vi "Parse Frequencies.vi"(0 "Frequencies in":string[](array[string]), 11 "error in (no error)":errorcluster) -> (4 "Frequencies out":dbl[](array[numeric]), 15 "error out":errorcluster)   [LabVIEW 2023, in "RFCalAndFixtureCharact.Common.lvlib"]
uses:
  RFCalAndFixtureCharact.Common.lvlib
  <vilib>/regexp/Match Regular Expression.xnode
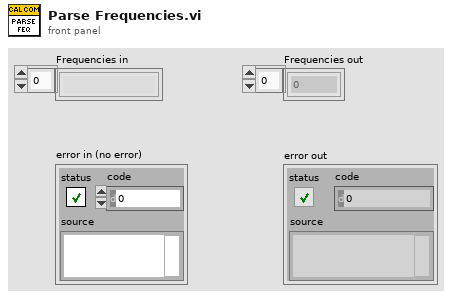
[diagram p1: front panel]
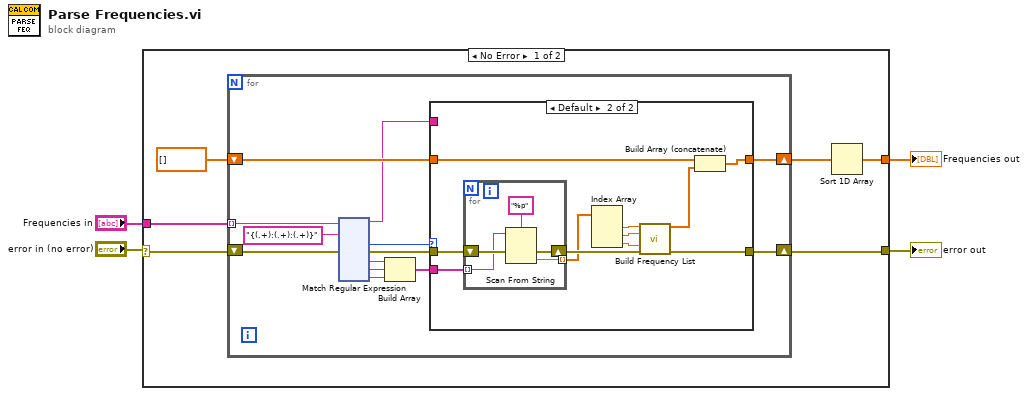
[diagram p0: block diagram]
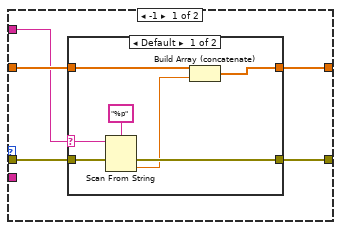
[diagram p2: hidden frame]
diagram:
  n1 = case shown="No Error" "error in (no error)" {
    selector: "error in (no error)" -> [w7 w175]
    tunnel: [w6 w175] -> w3
    tunnel: "Frequencies in" -> [w10 _]
    tunnel: [w8 _] -> w1
    frame No Error {
      n2 = for {
        tunnel: w10 -> [w23] mode=indexing
        shift-right: [w18] -> w6
        shift-left: w7 -> [w21]
        shift-right: [w16] -> w9
        shift-left: dbl[] [] ("Frequencies out") -> [w17]
        n3 = xnode "Match Regular Expression"("input string"=w23, "regular expression"="{(.+):(.+):(.+)}", "error in"=w21) -> ("before match"=w15:string, "offset past match"=w20:i32, "error out"=w19:errorcluster, "submatch 1"=w14:string, "submatch 2"=w13:string, "submatch 3"=w12:string)  [unwired: 3 in, 2 out]
        n4 = Build Array(w14, w13, w12) -> (w11:string[])
        n5 = case shown="Default" w20 {
          tunnel: w19 -> [w25 w44]
          tunnel: [w28 w46] -> w18
          tunnel: w17 -> [w27 w48]
          tunnel: [w26 w47] -> w16
          tunnel: w15 -> [w24 _]
          tunnel: w11 -> [_ w42]
          frame -1 {
            n6 = case shown="Default" w24 {
              selector: w24 -> [w31 _]
              tunnel: [w32 w36] -> w28
              tunnel: w27 -> [w35 w37]
              tunnel: [w34 w37] -> w26
              tunnel: w25 -> [w33 w36]
              frame Default {
                n7 = Scan From String(format string="%p", input string=w31, error in=w33) -> (error out=w32:errorcluster, output 1=w29:dbl)  [unwired: 2 in, 2 out]
                n8 = Build Array (concatenate)(w35, w29) -> (w34:dbl[])
              }
              frame "" {
              }
            }
          }
          frame Default {
            n9 = for {
              shift-right: [w51] -> w43
              shift-left: w44 -> [w52]
              tunnel: w42 -> [w50] mode=indexing
              tunnel: [w49] -> w41 mode=indexing
              n10 = Scan From String(format string="%p", input string=w50, error in=w52) -> (error out=w51:errorcluster, output 1=w49:dbl)  [unwired: 2 in, 2 out]
            }
            n11 = Index Array(array=w41) -> (element #1=w40:dbl, element #2=w39:dbl, element #3=w38:dbl)  [unwired: 3 in]
            n12 = call "Build Frequency List.vi"("start"=w40, "step"=w39, "stop"=w38, "error in (no error)"=w43) -> ("Frequency List"=w45:dbl[], "error out"=w46:errorcluster)  [unwired: 10 in]
            n13 = Build Array (concatenate)(w48, w45) -> (w47:dbl[])
          }
        }
      }
      n14 = Sort 1D Array(array=w9) -> (sorted array=w8:dbl[])
    }
    frame Error {
    }
  }
  "error out" <- w3
  "Frequencies out" <- w1
